vi "比较批次号关键字不同.vi"(8 "批次号":string, 9 "外购件名称":string, 10 "产品型号":string) -> (1 "关键字正确":bool, 3 "批次号 2":string)   [LabVIEW 2013]
panel:
  in  "error in (no error)":errorcluster
  out "error out":errorcluster
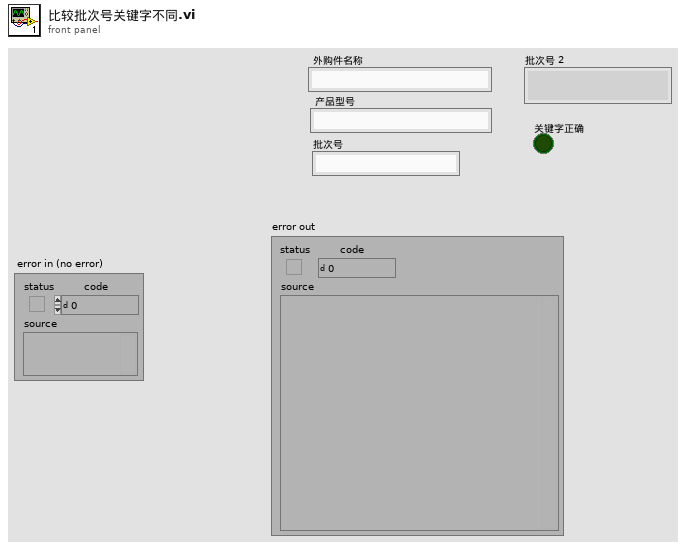
[diagram p1: front panel]
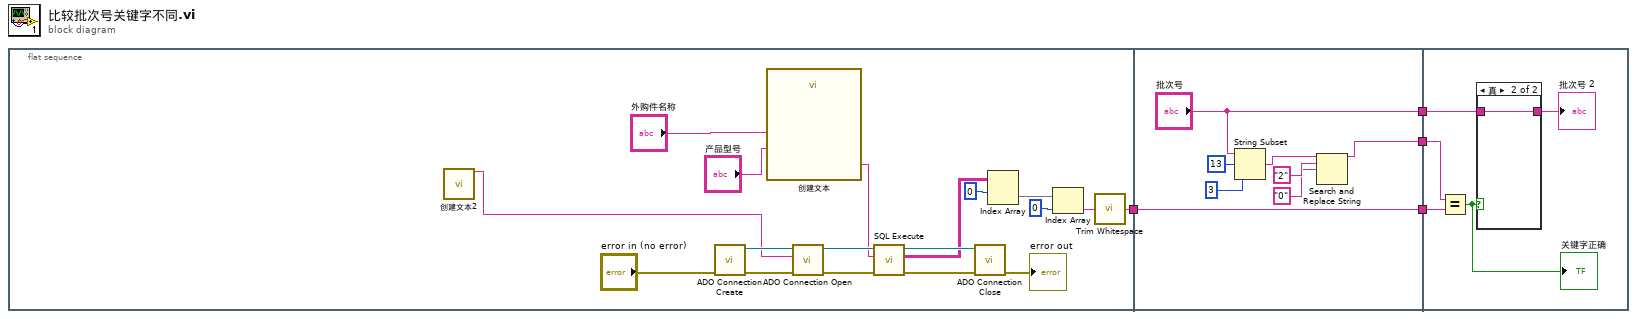
[diagram p0: block diagram]
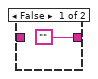
[diagram p2: hidden frame]
diagram:
  n1 = flat-sequence {
    tunnel: [w6] -> w3
    tunnel: [w25] -> w4
    tunnel: w3 -> [w30]
    tunnel: [w30] -> w2
    tunnel: ["批次号"] -> w1
    tunnel: w4 -> [w35]
    tunnel: w2 -> [w34]
    tunnel: w1 -> [w32]
    frame #0 {
      n2 = call "创建文本2"() -> ("Result"=w5:string)  [unwired: 14 in, 1 out]
      n3 = call "ADO Connection Create.vi"("error in (no error)"="error in (no error)") -> ("error out"=w21:errorcluster, "ADODB._Connection Out"=w22:refnum<k7>)  [unwired: 9 out]
      n4 = call "创建文本"("外购件名称"="外购件名称", "产品型号"="产品型号") -> ("Result"=w14:string)  [unwired: 12 in, 1 out]
      n5 = call "ADO Connection Open.vi"("error in (no error)"=w21, "ConnectionString"=w5, "ADODB._Connection In"=w22) -> ("error out"=w18:errorcluster, "ADODB._Connection Out"=w19:refnum<k7>)  [unwired: 7 out]
      n6 = call "SQL Execute.vi"("error in (no error)"=w18, "Command Text"=w14, "ADODB._Connection In"=w19) -> ("error out"=w16:errorcluster, "Data"=w11:string[][], "ADODB._Connection Out"=w17:refnum<k7>)  [unwired: 5 in, 1 out]
      n7 = call "ADO Connection Close.vi"("error in (no error)"=w16, "ADODB._Connection In"=w17) -> ("error out"=→"error out":errorcluster)  [unwired: 8 in, 1 out]
      n8 = Index Array(array=w11, index (row)=0 ("索引 (行)")) -> (element=w9:string[])  [unwired: 1 in]
      n9 = Index Array(array=w9, index=0 ("索引")) -> (element=w7:string)
      n10 = call <vilib>:"Trim Whitespace.vi"("string"=w7) -> ("trimmed string"=w6:string)  [unwired: 1 in]
    }
    frame #1 {
      n11 = String Subset(string="批次号", offset (0)=13 ("偏移量(0)"), length (rest)=3 ("长度（剩余）")) -> (substring=w26:string)
      n12 = Search and Replace String(input string=w26, search string="2" ("搜索字符串"), replace string="0" ("替换字符串(\"\")")) -> (result string=w25:string)  [unwired: 5 in, 3 out]
    }
    frame #2 {
      n13 = Equal?(x=w35, y=w34) -> (x = y?=w33:bool)
      "关键字正确" <- w33
      n14 = case shown="真" w33 {
        tunnel: w32 -> [_ w37]
        tunnel: ["" w37] -> w31
        frame False {
        }
        frame True {
        }
      }
      "批次号 2" <- w31
    }
  }
